vi "LVDeleteFile_Provider_OnCommand.vi"(10 "Command ID":string, 11 "objects":T1[](array[typedef])) -> ()   [LabVIEW 2018]
uses:
  <resource>/Framework/Providers/API/ItemRef.ctl
panel:
  out "error out":errorcluster
  in  "error in":errorcluster
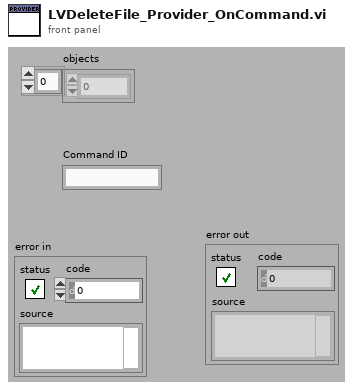
[diagram p1: front panel]
types:
  T1 = typedef "ItemRef.ctl" = u64
  T2 = enum16{"Left Button", "Center Button", "Right Button", "Window Close"}
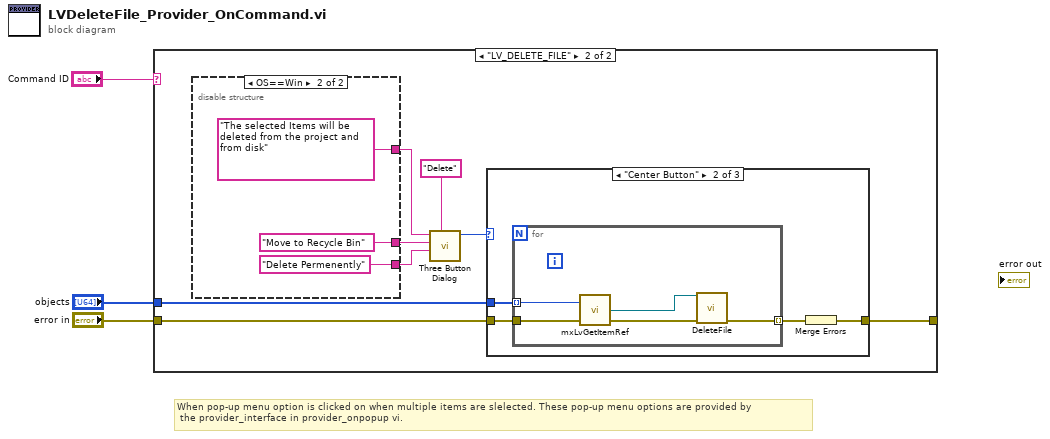
[diagram p0: block diagram]
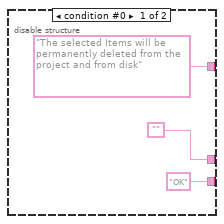
[diagram p3: hidden frame]
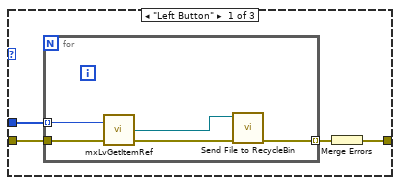
[diagram p4: hidden frame]
diagram:
  # "When pop-up menu option is clicked on when multiple items are slelected. These pop-up menu options are provided by\n the provider_interface in provider_onpopup vi."
  n1 = case shown="\"LV_DELETE_FILE\"" "Command ID" {
    tunnel: "error in" -> [w4 w12]
    tunnel: [w4 w11] -> _
    tunnel: "objects" -> [_ w10]
    frame Default {
    }
    frame "LV_DELETE_FILE" {
      n2 = disable-structure shown="OS==Win" {
        disable-tunnel: ["The selected Items will be permanently deleted from the project and from disk" ("message") "The selected Items will be deleted from the project and from disk" ("message")] -> w9
        disable-tunnel: ["" "Move to Recycle Bin" ("message")] -> w7
        disable-tunnel: ["OK" ("message") "Delete Permenently" ("message")] -> w6
        frame condition #0 {
        }
        frame condition #1 (active) {
        }
      }
      n3 = call <vilib>:"Three Button Dialog.vi"("Window Title (\"\")"="Delete" ("Window Title (\"\")"), "Center Button Text (\"No\")"=w6, "Left Button Text (\"Yes\")"=w7, "message"=w9) -> ("Which Button?"=w8:T2)  [unwired: 7 in]
      n4 = case shown="\"Center Button\"" w8 {
        tunnel: w10 -> [w22 w31 _]
        tunnel: w12 -> [w21 w30 w37]
        tunnel: [w19 w28 w37] -> w11
        frame "Left Button" {
          n5 = for {
            tunnel: w22 -> [w27] mode=indexing
            tunnel: w21 -> [w26]
            tunnel: [w23] -> w20 mode=indexing
            n6 = call <resource>:"mxLvGetItemRef.vi"("Item"=w27, "error in"=w26) -> ("Item Refnum"=w25:refnum<vi>, "error out"=w24:errorcluster)  [unwired: 1 out]
            n7 = call "Send File to RecycleBin.vi"("error in"=w24, "Item Refnum"=w25) -> ("error out"=w23:errorcluster)  [unwired: 9 in]
          }
          n8 = Merge Errors(w20) -> (w19:errorcluster)
        }
        frame "Center Button" {
          n9 = for {
            tunnel: w31 -> [w36] mode=indexing
            tunnel: w30 -> [w35]
            tunnel: [w34] -> w29 mode=indexing
            n10 = call <resource>:"mxLvGetItemRef.vi"("Item"=w36, "error in"=w35) -> ("Item Refnum"=w32:refnum<vi>, "error out"=w33:errorcluster)  [unwired: 1 out]
            n11 = call "DeleteFile.vi"("Item Refnum"=w32, "error in"=w33) -> ("error out"=w34:errorcluster)  [unwired: 13 in]
          }
          n12 = Merge Errors(w29) -> (w28:errorcluster)
        }
        frame Default {
        }
      }
    }
  }
